vi "timeoutMclksToMicroseconds.vi"(1 "vcsel_period_pclks":u8, 2 "timeout_period_mclks":u16) -> (0 "timeout_period_us":u32)   [LabVIEW 2018]
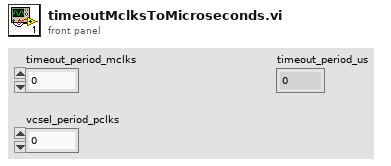
[diagram p1: front panel]
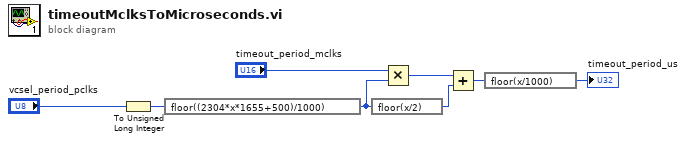
[diagram p0: block diagram]
diagram:
  n1 = To Unsigned Long Integer(number="vcsel_period_pclks") -> (unsigned 32bit integer=w8:u32)
  n2 = expression code="floor((2304*x*1655+500)/1000)"(w8) -> (w6:u32)
  n3 = expression code="floor(x/2)"(w6) -> (w5:u32)
  n4 = Multiply(x="timeout_period_mclks", y=w6) -> (x*y=w7:u32)
  n5 = Add(x=w7, y=w5) -> (x+y=w4:u32)
  n6 = expression code="floor(x/1000)"(w4) -> (→"timeout_period_us":u32)
